vi "BGP - Data - Capacitance.vi"(8 "error in":errorcluster) -> (0 "error out":errorcluster)   [LabVIEW 2012]
uses:
  Controls/Object Ref and Name.ctl
  Controls/Global Stop States.ctl
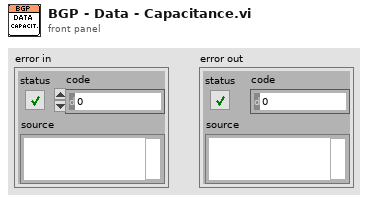
[diagram p1: front panel]
types:
  T1 = typedef "Object Ref and Name.ctl" = cluster{"Name":string, "Reference":refnum<vi>}
  T2 = typedef "Global Stop States.ctl" = enum16{"STOP", "STATUS", "INIT"}
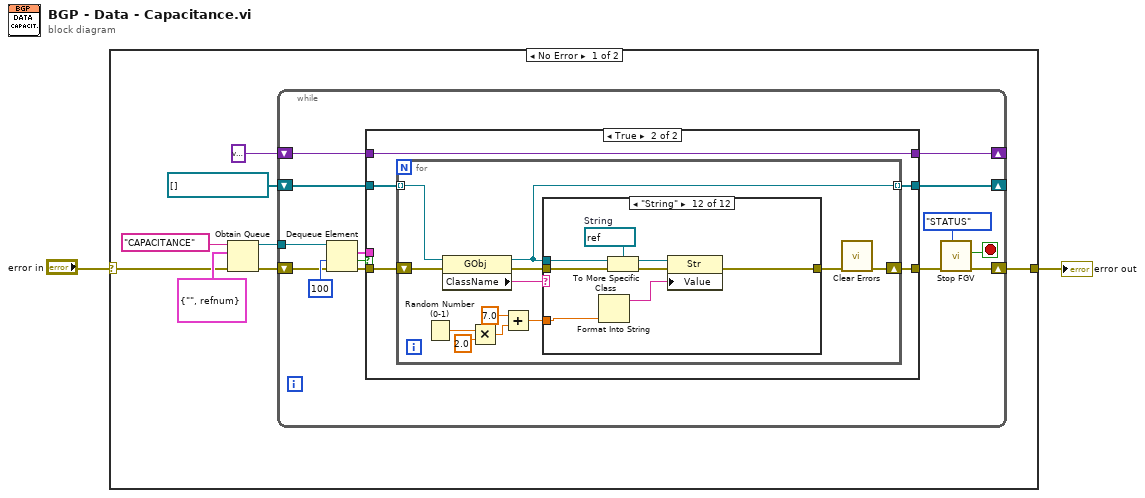
[diagram p0: block diagram]
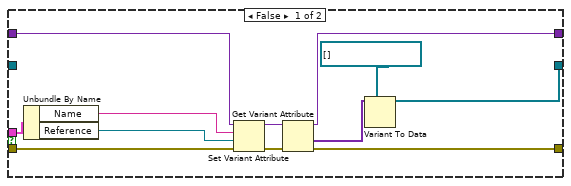
[diagram p2: hidden frame]
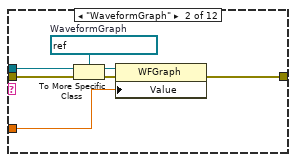
[diagram p4: hidden frame]
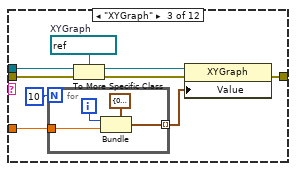
[diagram p5: hidden frame]
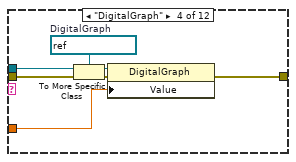
[diagram p6: hidden frame]
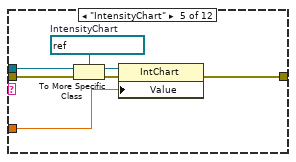
[diagram p7: hidden frame]
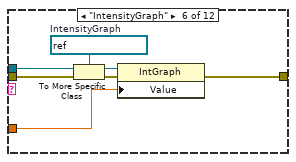
[diagram p8: hidden frame]
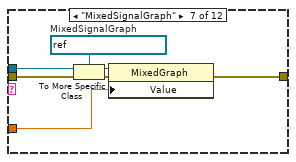
[diagram p9: hidden frame]
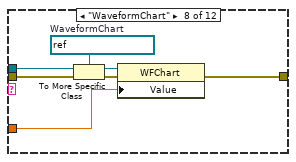
[diagram p10: hidden frame]
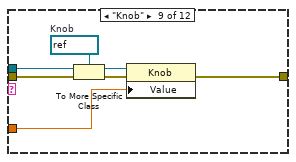
[diagram p11: hidden frame]
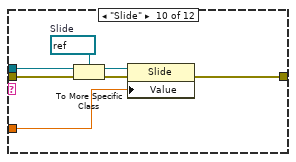
[diagram p12: hidden frame]
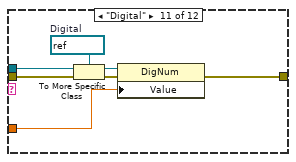
[diagram p13: hidden frame]
diagram:
  n1 = case shown="No Error" "error in" {
    selector: "error in" -> [w3 w139]
    tunnel: [w10 w139] -> w2
    frame No Error {
      n2 = Obtain Queue(name (unnamed)="CAPACITANCE", element data type=T1 {"Name"="", "Reference"=refnum}, error in (no error)=w3) -> (queue out=w9:refnum<queue>, error out=w5:errorcluster)  [unwired: 2 in, 1 out]
      n3 = while {
        tunnel: w9 -> [w24]
        shift-right: [w20] -> _
        shift-left: variant ("variant") -> [w22]
        shift-right: [w14] -> w10
        shift-left: w5 -> [w18]
        shift-right: [w17] -> _
        shift-left: refnum<vi>[] [] -> [w16]
        stop <- w11 stop-if-true
        n4 = Dequeue Element(queue=w24, timeout in ms (-1)=100, error in (no error)=w18) -> (element=w21:T1, timed out?=w15:bool, error out=w19:errorcluster)  [unwired: 1 out]
        n5 = case shown="True" w15 {
          tunnel: w22 -> [w36 w41]
          tunnel: w21 -> [w35 _]
          tunnel: [w31 w41] -> w20
          tunnel: w19 -> [w30 w40]
          tunnel: [w28 w37] -> w13
          tunnel: [w25 w38] -> w17
          tunnel: w16 -> [_ w39]
          frame False {
            n6 = Unbundle By Name(w35) -> ("Name"=w34:string, "Reference"=w33:refnum<vi>)
            n7 = Set Variant Attribute(Variant=w36, name=w34, value=w33, error in=w30) -> (Variant out=w32:variant, error out=w29:errorcluster)  [unwired: 1 out]
            n8 = Get Variant Attribute(Variant=w32, error in=w29) -> (duplicate Variant=w31:variant, values=w26:variant[], error out=w28:errorcluster)  [unwired: 2 in, 1 out]
            n9 = Variant To Data(type=refnum<vi>[] [], Variant=w26) -> (data=w25:refnum<vi>[])  [unwired: 1 in, 1 out]
          }
          frame True {
            n10 = for {
              tunnel: w39 -> [w49] mode=indexing
              shift-right: [w45] -> w37
              shift-left: w40 -> [w47]
              tunnel: [w48] -> w38 mode=indexing
              n11 = Random Number (0-1)() -> (number: 0 to 1=w53:dbl)
              n12 = property class="GObj"(reference=w49, error in=w47) -> (reference out=w48:refnum<vi>, error out=w46:errorcluster, "ClassName"=w43:string)
              n13 = Multiply(x=w53, y=2.0) -> (x*y=w42:dbl)
              n14 = Add(x=7.0 ("y"), y=w42) -> (x+y=w50:dbl)
              n15 = case shown="\"String\"" w43 {
                tunnel: w50 -> [_ w59 w62 w79 w86 w93 w100 w107 w114 w121 w128 w132]
                tunnel: w48 -> [_ w58 w68 w78 w85 w92 w99 w106 w113 w120 w127 w136]
                tunnel: w46 -> [w54 w56 w66 w76 w83 w90 w97 w104 w111 w118 w125 w134]
                tunnel: [w54 w57 w67 w77 w84 w91 w98 w105 w112 w119 w126 w135] -> w44
                frame "False", Default {
                }
                frame "WaveformGraph" {
                  w61 = refnum<vi> refnum  # WaveformGraph
                  n16 = To More Specific Class(target class=w61, reference=w58, error in=w56) -> (specific class reference=w60:refnum<vi>, error out=w55:errorcluster)
                  n17 = property class="WFGraph"(reference=w60, error in=w55, "Value"=w59) -> (error out=w57:errorcluster)  [unwired: 1 out]
                }
                frame "XYGraph" {
                  w70 = refnum<vi> refnum  # XYGraph
                  n18 = for {
                    N: 10 -> [_]
                    tunnel: [w73] -> w63 mode=indexing
                    tunnel: w62 -> [w71]
                    i -> [w72]
                    n19 = Bundle(cluster=cluster{dbl, dbl} {0.0, 0.0}, w72, w71) -> (w73:cluster{dbl, dbl})
                  }
                  n20 = To More Specific Class(target class=w70, reference=w68, error in=w66) -> (specific class reference=w69:refnum<vi>, error out=w65:errorcluster)
                  n21 = property class="XYGraph"(reference=w69, error in=w65, "Value"=w63) -> (error out=w67:errorcluster)  [unwired: 1 out]
                }
                frame "DigitalGraph" {
                  w81 = refnum<vi> refnum  # DigitalGraph
                  n22 = To More Specific Class(target class=w81, reference=w78, error in=w76) -> (specific class reference=w80:refnum<vi>, error out=w75:errorcluster)
                  n23 = property class="DigitalGraph"(reference=w80, error in=w75, "Value"=w79) -> (error out=w77:errorcluster)  [unwired: 1 out]
                }
                frame "IntensityChart" {
                  w88 = refnum<vi> refnum  # IntensityChart
                  n24 = To More Specific Class(target class=w88, reference=w85, error in=w83) -> (specific class reference=w87:refnum<vi>, error out=w82:errorcluster)
                  n25 = property class="IntChart"(reference=w87, error in=w82, "Value"=w86) -> (error out=w84:errorcluster)  [unwired: 1 out]
                }
                frame "IntensityGraph" {
                  w95 = refnum<vi> refnum  # IntensityGraph
                  n26 = To More Specific Class(target class=w95, reference=w92, error in=w90) -> (specific class reference=w94:refnum<vi>, error out=w89:errorcluster)
                  n27 = property class="IntGraph"(reference=w94, error in=w89, "Value"=w93) -> (error out=w91:errorcluster)  [unwired: 1 out]
                }
                frame "MixedSignalGraph" {
                  w102 = refnum<vi> refnum  # MixedSignalGraph
                  n28 = To More Specific Class(target class=w102, reference=w99, error in=w97) -> (specific class reference=w101:refnum<vi>, error out=w96:errorcluster)
                  n29 = property class="MixedGraph"(reference=w101, error in=w96, "Value"=w100) -> (error out=w98:errorcluster)  [unwired: 1 out]
                }
                frame "WaveformChart" {
                  w109 = refnum<vi> refnum  # WaveformChart
                  n30 = To More Specific Class(target class=w109, reference=w106, error in=w104) -> (specific class reference=w108:refnum<vi>, error out=w103:errorcluster)
                  n31 = property class="WFChart"(reference=w108, error in=w103, "Value"=w107) -> (error out=w105:errorcluster)  [unwired: 1 out]
                }
                frame "Knob" {
                  w116 = refnum<vi> refnum  # Knob
                  n32 = To More Specific Class(target class=w116, reference=w113, error in=w111) -> (specific class reference=w115:refnum<vi>, error out=w110:errorcluster)
                  n33 = property class="Knob"(reference=w115, error in=w110, "Value"=w114) -> (error out=w112:errorcluster)  [unwired: 1 out]
                }
                frame "Slide" {
                  w123 = refnum<vi> refnum  # Slide
                  n34 = To More Specific Class(target class=w123, reference=w120, error in=w118) -> (specific class reference=w122:refnum<vi>, error out=w117:errorcluster)
                  n35 = property class="Slide"(reference=w122, error in=w117, "Value"=w121) -> (error out=w119:errorcluster)  [unwired: 1 out]
                }
                frame "Digital" {
                  w130 = refnum<vi> refnum  # Digital
                  n36 = To More Specific Class(target class=w130, reference=w127, error in=w125) -> (specific class reference=w129:refnum<vi>, error out=w124:errorcluster)
                  n37 = property class="DigNum"(reference=w129, error in=w124, "Value"=w128) -> (error out=w126:errorcluster)  [unwired: 1 out]
                }
                frame "String" {
                  w138 = refnum<vi> refnum  # String
                  n38 = Format Into String(w132) -> (resulting string=w131:string)  [unwired: 3 in, 1 out]
                  n39 = To More Specific Class(target class=w138, reference=w136, error in=w134) -> (specific class reference=w137:refnum<vi>, error out=w133:errorcluster)
                  n40 = property class="Str"(reference=w137, error in=w133, "Value"=w131) -> (error out=w135:errorcluster)  [unwired: 1 out]
                }
              }
              n41 = call <vilib>:"Clear Errors.vi"("error in (no error)"=w44) -> ("error out"=w45:errorcluster)  [unwired: 6 in]
            }
          }
        }
        n42 = call "Stop FGV.vi"("Operation In"=Global_Stop_States."STATUS", "error in"=w13) -> ("error out"=w14:errorcluster, "Stop?"=w11:bool)  [unwired: 8 in]
      }
    }
    frame Error {
    }
  }
  "error out" <- w2
